vi "Valid Row Column or Not.vi"(8 "error in (no error)":errorcluster, 9 "cursor position in":cluster{"row":i8, "column":i8}, 11 "cluster of private data in":T1={"FPGA VI Reference"=refnum, "device index"=0, "screen size"=enum."8x1", "font size"=enum."5x8", "auto wrap"=FALSE, "alignment"=enum."None", "number of line"=enum."2 lines", "shift 0"=0, "entry mode 0"=enum."increment & no shift", "shift 1"=0, "entry mode 1"=enum."increment & no shift"}) -> (0 "error out":errorcluster, 1 "cursor position out":cluster{"row":i8, "column":i8}, 3 "cluster of private data out":T1={"FPGA VI Reference"=refnum, "device index"=0, "screen size"=enum."8x1", "font size"=enum."5x8", "auto wrap"=FALSE, "alignment"=enum."None", "number of line"=enum."2 lines", "shift 0"=0, "entry mode 0"=enum."increment & no shift", "shift 1"=0, "entry mode 1"=enum."increment & no shift"})   [LabVIEW 2017, in "HD44780.lvclass"]
uses:
  HD44780.lvclass
  Common/HD44780 Common.lvlib
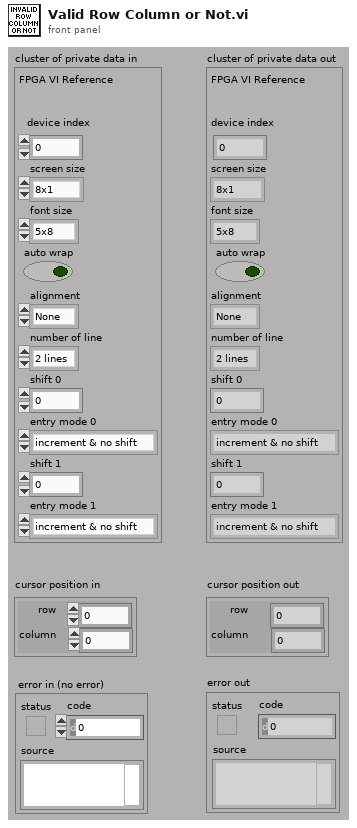
[diagram p1: front panel]
types:
  T1 = cluster{"FPGA VI Reference":refnum<k20>, "device index":i8, "screen size":enum8{"8x1", "8x2", "12x4", "16x1", "16x2", "16x4", "20x1", "20x2", "20x4", "24x1", "24x2", "40x2", "40x4"}, "font size":enum8{"5x8", "5x10"}, "auto wrap":bool, "alignment":enum16{"None", "Left", "Center", "Right"}, "number of line":enum8{"1 line", "2 lines"}, "shift 0":i8, "entry mode 0":enum8{"increment & no shift", "increment & shift", "decrement & no shift", "decrement & shift"}, "shift 1":i8, "entry mode 1":enum8{"increment & no shift", "increment & shift", "decrement & no shift", "decrement & shift"}}
  T2 = enum8{"8x1", "8x2", "12x4", "16x1", "16x2", "16x4", "20x1", "20x2", "20x4", "24x1", "24x2", "40x2", "40x4"}
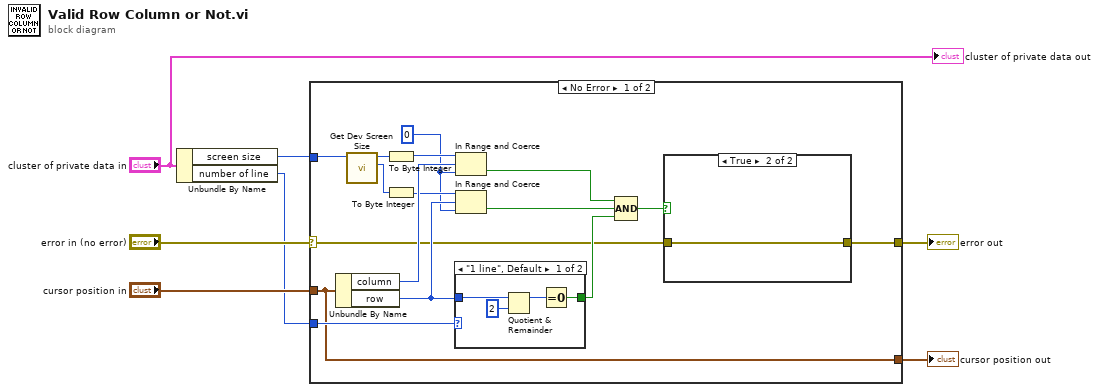
[diagram p0: block diagram]
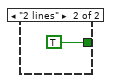
[diagram p2: hidden frame]
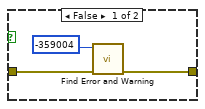
[diagram p3: hidden frame]
diagram:
  n1 = Unbundle By Name("cluster of private data in") -> ("screen size"=w3:T2, "number of line"=w2:enum8{"1 line", "2 lines"})
  n2 = case shown="No Error" "error in (no error)" {
    selector: "error in (no error)" -> [w8 w33]
    tunnel: [w23 w33] -> w6
    tunnel: w3 -> [w20 _]
    tunnel: "cursor position in" -> [w9 _]
    tunnel: w2 -> [w19 _]
    tunnel: [w9 _] -> w1
    frame No Error {
      w14 = i8 0 ("lower limit")
      n3 = Unbundle By Name(w9) -> ("column"=w17:i8, "row"=w15:i8)
      n4 = call "Get Dev Screen Size.vi"("screen size"=w20) -> ("Max Row number"=w21:u8, "Max Column number"=w22:u8)  [unwired: 9 in]
      n5 = To Byte Integer(number=w22) -> (8bit integer=w18:i8)
      n6 = To Byte Integer(number=w21) -> (8bit integer=w16:i8)
      n7 = case shown="\"1 line\", Default" w19 {
        tunnel: w15 -> [w27 _]
        tunnel: [w25 TRUE] -> w11
        frame "1 line", Default {
          n8 = Quotient & Remainder(x=w27, y=i8 2) -> (x-y*floor(x/y)=w26:i8)  [unwired: 1 out]
          n9 = Equal To 0?(x=w26) -> (x = 0?=w25:bool)
        }
        frame "2 lines" {
        }
      }
      n10 = In Range and Coerce(upper limit=w18, x=w17, lower limit=w14) -> (In Range?=w13:bool)  [unwired: 1 out]
      n11 = In Range and Coerce(upper limit=w16, x=w15, lower limit=w14) -> (In Range?=w12:bool)  [unwired: 1 out]
      n12 = Compound Arithmetic op=AND(w13, w12, w11) -> (w10:bool)
      n13 = case shown="True" w10 {
        tunnel: [w31 w32] -> w23
        tunnel: w8 -> [w29 w32]
        frame False {
          n14 = call "Find Error and Warning.vi"("error in (no error)"=w29, "error code"=-359004) -> ("error out"=w31:errorcluster)  [unwired: 9 in]
        }
        frame True {
        }
      }
    }
    frame Error {
    }
  }
  "error out" <- w6
  "cursor position out" <- w1
  "cluster of private data out" <- "cluster of private data in"
